vi "Get Daily Timestamps for Feb.vi"() -> (1 "To":timestamp[](array[timestamp]), 2 "From":timestamp[](array[timestamp]))   [LabVIEW 2020, in "Data Manager.lvclass"]
uses:
  Data Manager.lvclass
panel:
  in  "Number of Days":i32=28
  in  "Time Stamp":timestamp=timestamp(3694986000 s since 1904-01-01)
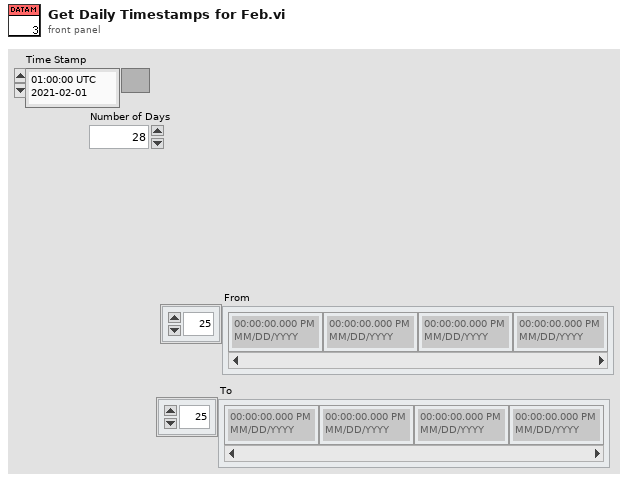
[diagram p1: front panel]
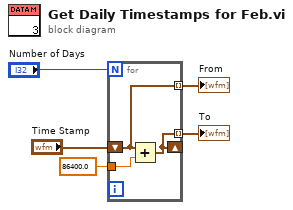
[diagram p0: block diagram]
diagram:
  n1 = for {
    N: "Number of Days" -> [_]
    tunnel: 86400.0 -> [w8]
    tunnel: [w6] -> w1 mode=indexing
    tunnel: [w7] -> w2 mode=indexing
    shift-right: [w6] -> _
    shift-left: "Time Stamp" -> [w7]
    n2 = Add(x=w7, y=w8) -> (x+y=w6:timestamp)
  }
  "From" <- w2
  "To" <- w1
